vi "op_rel_v1.vi"() -> ()   [LabVIEW 2009]
panel:
  in  "Knob":u8(knob) scale=0.0..9.0
  out "L":bool
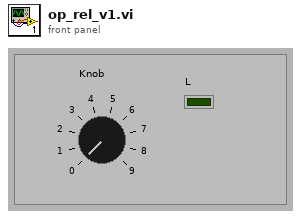
[diagram p1: front panel]
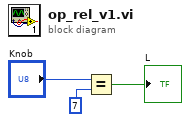
[diagram p0: block diagram]
diagram:
  n1 = Equal?(x="Knob", y=7) -> (x = y?=→"L":bool)
